vi "item selection new tree.vi"(8 "error in (no error)":errorcluster, 11 "Tree ref":refnum<vi>) -> (0 "error out":errorcluster, 3 "Loop data":T1)   [LabVIEW 2020, in "UI_ItemSelect_OpenSource.lvlib"]
uses:
  UI_ItemSelect_OpenSource.lvlib
  Tree item select loop data.ctl
  Item select ref type.ctl
  Tree item loop data.ctl
  Tree item selection indices.ctl
  checkbox state.ctl
  item select tree lock states.ctl
  <vilib>/picture/picture.llb/imagedata.ctl
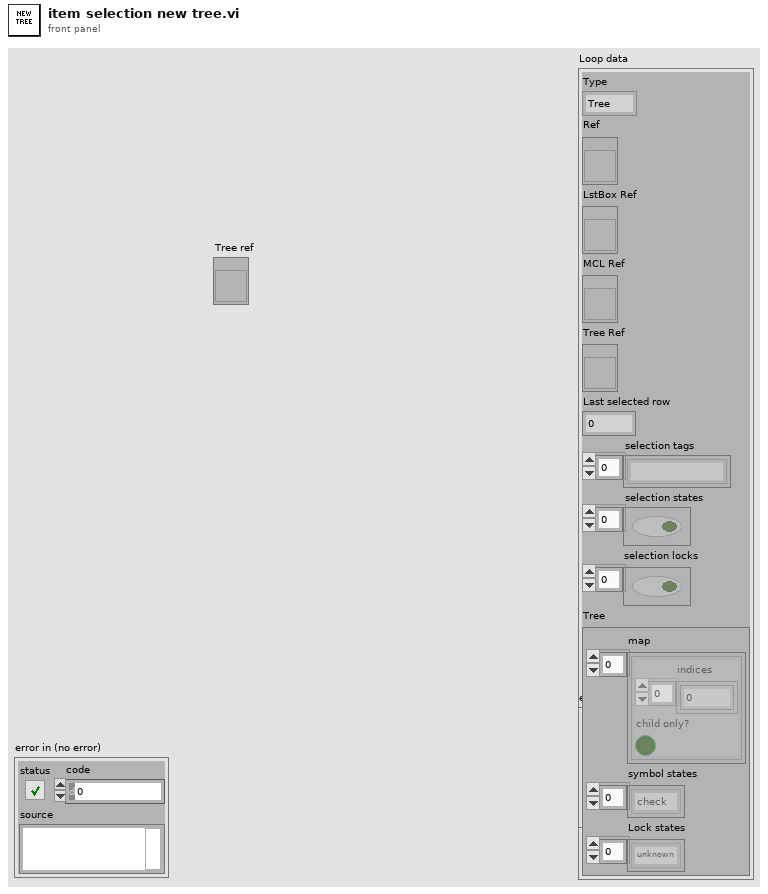
[diagram p1: front panel]
types:
  T1 = typedef "UI_ItemSelect_OpenSource.lvlib/Tree item select loop data.ctl" = cluster{"Type":T2, "Ref":refnum<vi>, "LstBox Ref":refnum<vi>, "MCL Ref":refnum<vi>, "Tree Ref":refnum<vi>, "Last selected row":i32, "selection tags":string[], "selection states":bool[], "selection locks":bool[], "Tree":T3}
  T2 = typedef "UI_ItemSelect_OpenSource.lvlib/Item select ref type.ctl" = enum16{"Tree", "MCL", "ListBox"}
  T3 = typedef "UI_ItemSelect_OpenSource.lvlib/Tree item loop data.ctl" = cluster{"map":T4[], "symbol states":T5[], "Lock states":T6[]}
  T4 = typedef "UI_ItemSelect_OpenSource.lvlib/Tree item selection indices.ctl" = cluster{"indices":i32[], "child only?":bool}
  T5 = typedef "UI_ItemSelect_OpenSource.lvlib/checkbox state.ctl" = enum16{"unknown", "check", "some", "no check"}
  T6 = typedef "UI_ItemSelect_OpenSource.lvlib/item select tree lock states.ctl" = enum16{"unknown", "locked", "unlocked"}
  T7 = typedef "imagedata.ctl" = cluster{"image type":i32, "image depth":i32, "image":u8[], "mask":u8[], "colors":u32[], "Rectangle":cluster{"left":i16, "top":i16, "right":i16, "bottom":i16}}
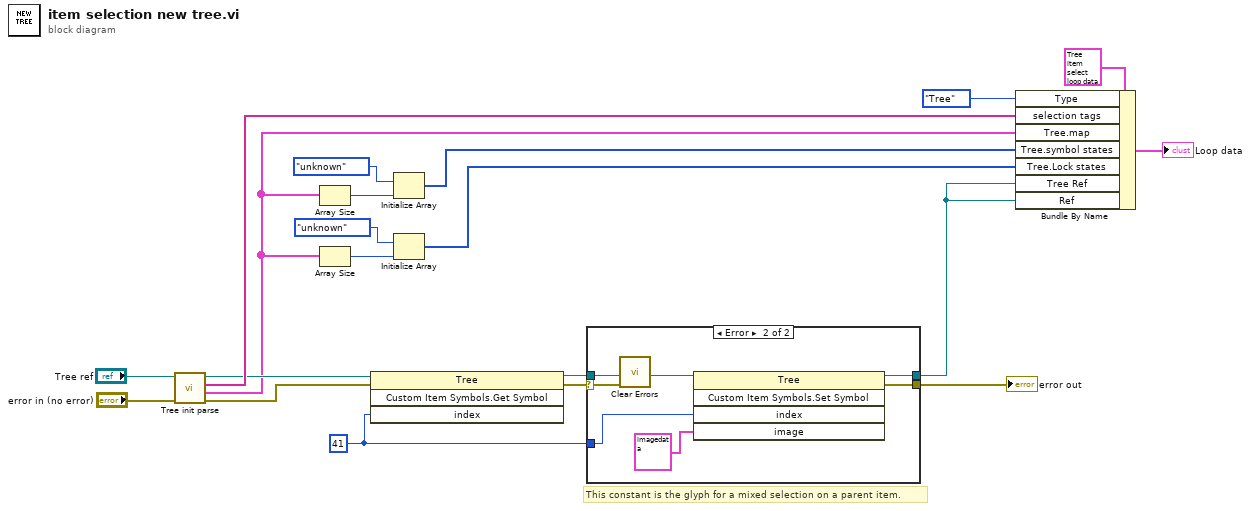
[diagram p0: block diagram]
diagram:
  w9 = 41 ("Index")
  # "This constant is the glyph for a mixed selection on a parent item."
  n1 = call "Tree init parse.vi"("error in (no error)"="error in (no error)", "Tree ref"="Tree ref") -> ("error out"=w8:errorcluster, "map"=w3:T4[], "Selection Tags"=w14:string[], "Tree ref"=w12:refnum<vi>)  [unwired: 6 in]
  n2 = Array Size(array=w3) -> (size(s)=w18:i32)
  n3 = Array Size(array=w3) -> (size(s)=w4:i32)
  n4 = invoke class="Tree" method="Custom Item Symbols.Get Symbol"(reference=w12, error in=w8, "index"=w9) -> (reference out=w10:refnum<vi>, error out=w11:errorcluster)  [unwired: 1 in, 2 out]
  n5 = Initialize Array(checkbox_state."unknown", w18) -> (w16:T5[])
  n6 = Initialize Array(item_select_tree_lock_states."unknown", w4) -> (w2:T6[])
  n7 = case shown="Error" w11 {
    selector: w11 -> [w21 w23]
    tunnel: [w22 w28] -> w5
    tunnel: [w21 w27] -> w7
    tunnel: w10 -> [w22 w25]
    tunnel: w9 -> [_ w24]
    frame No Error {
    }
    frame Error {
      n8 = call <vilib>:"Clear Errors.vi"("error in (no error)"=w23) -> ()  [unwired: 5 in, 2 out]
      n9 = invoke class="Tree" method="Custom Item Symbols.Set Symbol"(reference=w25, "index"=w24, "image"=T7 {"image type"=0, "image depth"=24, "image"=[142, 143, 143, 142, 143, 143, 142, 143, 143, 142, 143, 143, 142, 143, 143, 142, 143, 143, 142, 143, 143, 142, 143, 143, 142, 143, 143, 142, 143, 143, 142, 143, 143, 142, 143, 143, 142, 143, 143, 142, 143, 143, 244, 244, 244, 244, 244, 244, 244, 244, 244, 244, 244, 244, 244, 244, 244, 244, 244, 244, 244, 244, 244, 244, 244, 244, 244, 244, 244, 244, 244, 244, 244, 244, 244, 142, 143, 143, 142, 143, 143, 244, 244, 244, 41, 98, 141, 42, 98, 142, 42, 98, 142, 42, 98, 141, 41, 97, 140, 40, 96, 138, 40, 94, 135, 39, 91, 132, 38, 89, 128, 244, 244, 244, 142, 143, 143, 142, 143, 143, 244, 244, 244, 41, 98, 141, 127, 200, 228, 123, 195, 225, 117, 190, 221, 110, 183, 217, 104, 175, 211, 96, 167, 204, 89, 157, 196, 36, 86, 124, 244, 244, 244, 142, 143, 143, 142, 143, 143, 244, 244, 244, 41, 97, 139, 123, 194, 224, 47, 168, 213, 47, 166, 211, 46, 164, 208, 45, 159, 203, 43, 153, 197, 80, 146, 187, 35, 82, 118, 244, 244, 244, 142, 143, 143, 142, 143, 143, 244, 244, 244, 40, 95, 137, 116, 187, 218, 46, 164, 209, 45, 162, 206, 44, 157, 201, 43, 151, 194, 41, 145, 187, 71, 134, 177, 32, 76, 110, 244, 244, 244, 142, 143, 143, 142, 143, 143, 244, 244, 244, 39, 93, 133, 109, 179, 212, 44, 158, 201, 43, 153, 196, 42, 147, 190, 40, 141, 183, 37, 133, 174, 62, 121, 166, 30, 70, 101, 244, 244, 244, 142, 143, 143, 142, 143, 143, 244, 244, 244, 38, 90, 129, 102, 169, 203, 42, 148, 191, 40, 142, 184, 38, 135, 176, 36, 127, 167, 34, 119, 159, 52, 107, 154, 27, 64, 92, 244, 244, 244, 142, 143, 143, 142, 143, 143, 244, 244, 244, 36, 85, 123, 93, 157, 194, 39, 137, 179, 36, 129, 170, 34, 120, 160, 31, 111, 150, 30, 105, 143, 44, 96, 143, 25, 59, 85, 244, 244, 244, 142, 143, 143, 142, 143, 143, 244, 244, 244, 35, 81, 117, 85, 146, 184, 76, 134, 174, 68, 122, 164, 59, 110, 153, 50, 101, 147, 44, 95, 143, 37, 89, 140, 25, 59, 85, 244, 244, 244, 142, 143, 143, 142, 143, 143, 244, 244, 244, 33, 78, 113, 31, 73, 106, 29, 68, 97, 26, 62, 89, 25, 59, 85, 25, 59, 85, 25, 58, 85, 25, 58, 85, 25, 59, 85, 244, 244, 244, 142, 143, 143, 142, 143, 143, 244, 244, 244, 244, 244, 244, 244, 244, 244, 244, 244, 244, 244, 244, 244, 244, 244, 244, 244, 244, 244, 244, 244, 244, 244, 244, 244, 244, 244, 244, 244, 244, 244, 142, 143, 143, 142, 143, 143, 142, 143, 143, 142, 143, 143, 142, 143, 143, 142, 143, 143, 142, 143, 143, 142, 143, 143, 142, 143, 143, 142, 143, 143, 142, 143, 143, 142, 143, 143, 142, 143, 143, 142, 143, 143], "mask"=[], "colors"=[], "Rectangle"={"left"=0, "top"=0, "right"=13, "bottom"=13}} ("image data")) -> (reference out=w28:refnum<vi>, error out=w27:errorcluster)  [unwired: 2 in, 3 out]
    }
  }
  "error out" <- w7
  n10 = Bundle By Name(cluster=T1 {"Type"=enum."Tree", "Ref"=refnum, "LstBox Ref"=refnum, "MCL Ref"=refnum, "Tree Ref"=refnum, "Last selected row"=0, "selection tags"=[], "selection states"=[], "selection locks"=[], "Tree"={"map"=[], "symbol states"=[], "Lock states"=[]}} ("Loop data"), "Type"=Item_select_ref_type."Tree", "selection tags"=w14, "Tree.map"=w3, "Tree.symbol states"=w16, "Tree.Lock states"=w2, "Tree Ref"=w5, "Ref"=w5) -> (→"Loop data":T1)
